vi "VIC_glb.vi"() -> ()   [LabVIEW 2018]
panel:
  in  "Scan Line":u16
  in  "Raster Line":u16
  in  "IRQ reg":u8
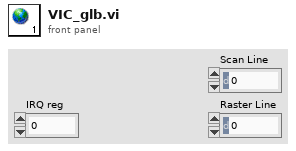
[diagram p1: front panel]
diagram:
